vi "GetNextFloat.vi"(11 "read buffer in":string) -> (2 "remaining string":string, 3 "Grabbed float":dbl)   [LabVIEW 2020]
panel:
  out "substring":string
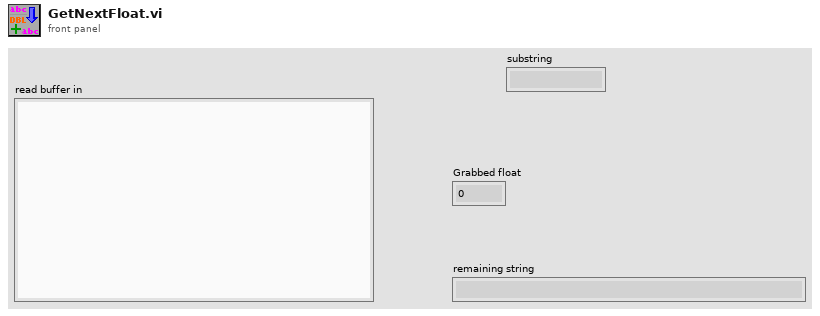
[diagram p1: front panel]
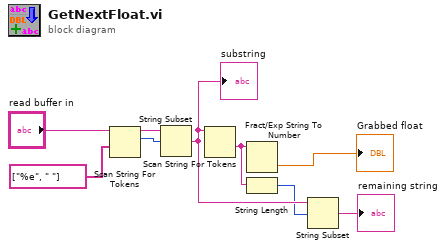
[diagram p0: block diagram]
diagram:
  n1 = Scan String For Tokens(7:string[] ["%e", " "] ("delimiters (\\s,\\t,\\r,\\n)"), 9:"read buffer in") -> (2:w4:i32, 3:w7:string)  [unwired: 4 in, 2 out]
  n2 = String Subset(string=w7, offset (0)=w4) -> (substring=w3:string)  [unwired: 1 in]
  "substring" <- w3
  n3 = Scan String For Tokens(9:w3) -> (1:w5:string)  [unwired: 5 in, 3 out]
  n4 = Fract/Exp String To Number(string=w5) -> (number=→"Grabbed float":dbl)  [unwired: 3 in, 1 out]
  n5 = String Length(string=w5) -> (length=w2:i32)
  n6 = String Subset(string=w3, offset (0)=w2) -> (substring=→"remaining string":string)  [unwired: 1 in]
